vi "AutoSteerAngle.vi"(4 "CurrentSteerAngle":dbl, 6 "CurrentDirection":dbl, 8 "Ycurrent":dbl, 9 "Xcurrent":dbl, 10 "Ywaypoint":dbl, 11 "Xwaypoint":dbl) -> (2 "NewSteerAngle":dbl)   [LabVIEW 2012]
doc: "This VI calculates steering angle from current robot position to next waypoint."
uses:
  <vilib>/addons/control/pid/pid.llb/PID (DBL).vi
  <vilib>/addons/control/pid/NI_PID_pid.lvlib
panel:
  in  "reinitialize? (F)":bool
  out "reranged":dbl
  out "SetpointCommand":dbl
  out "Waveform Chart 2":cluster{dbl, dbl}(graph)
  out "output range":cluster{"output high":dbl, "output low":dbl}={"output high"=100.0, "output low"=-100.0} {"output low" format="%.2f"; "output high" format="%.2f"}
  out "PID gains":T1={"proportional gain (Kc)"=20.0, "integral time (Ti, min)"=0.008, "derivative time (Td, min)"=0.001} {"derivative time (Td, min)" step=1e-05 format="%.5f"; "integral time (Ti, min)" step=0.0001 format="%.4f"; "proportional gain (Kc)" step=0.001 format="%.4f"}
  out "Waveform Chart":cluster{dbl, "CurrentDirection":dbl}(graph)
  out "towaypoint":dbl
  # "This Vi calculates sttering angle \nfrom current position to \nnext waypoint"
  # "0.120\n1.600\n0000"
  # "in degreees"
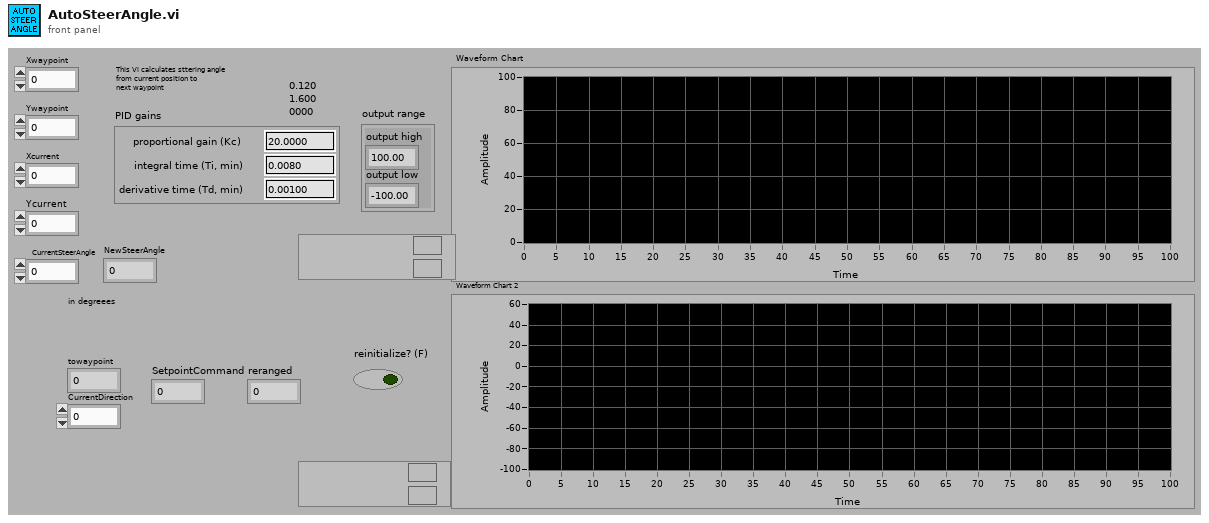
[diagram p1: front panel]
types:
  T1 = cluster{"proportional gain (Kc)":dbl, "integral time (Ti, min)":dbl, "derivative time (Td, min)":dbl}
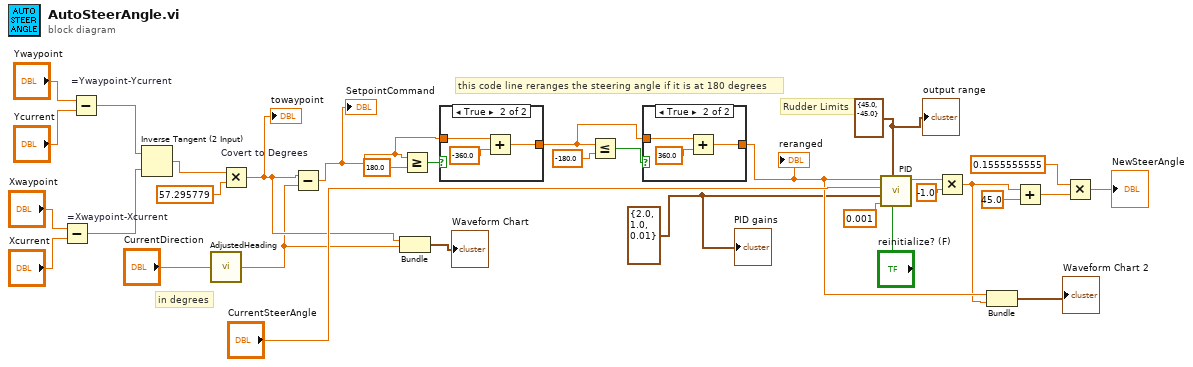
[diagram p0: block diagram]
diagram:
  w7 = T1 {"proportional gain (Kc)"=2.0, "integral time (Ti, min)"=1.0, "derivative time (Td, min)"=0.01} ("PID gains")
  w21 = cluster{"output high":dbl, "output low":dbl} {"output high"=45.0, "output low"=-45.0} ("output range")
  # "this code line reranges the steering angle if it is at 180 degrees"
  # "Rudder Limits"
  # "in degrees"
  n1 = Subtract "=Xwaypoint-Xcurrent"(x="Xwaypoint", y="Xcurrent") -> (x-y=w27:dbl)
  n2 = Subtract "=Ywaypoint-Ycurrent"(x="Ywaypoint", y="Ycurrent") -> (x-y=w28:dbl)
  n3 = Inverse Tangent (2 Input)(1:w27, 2:w28) -> (0:w25:dbl)
  n4 = call "AdjustedHeading.vi"("Heading In"="CurrentDirection") -> ("Heading Out"=w1:dbl)
  n5 = Multiply "Covert to Degrees"(x=w25, y=57.295779) -> (x*y=w13:dbl)
  "towaypoint" <- w13
  n6 = Subtract(x=w13, y=w1) -> (x-y=w17:dbl)
  "SetpointCommand" <- w17
  n7 = Bundle(w13, "Heading Out"=w1) -> (→"Waveform Chart":cluster{dbl, "Heading Out":dbl})  [unwired: 1 in]
  n8 = Greater Or Equal?(x=w17, y=180.0) -> (x >= y?=w18:bool)
  n9 = case shown="True" w18 {
    tunnel: w17 -> [w33 w36]
    tunnel: [w33 w34] -> w14
    frame False {
    }
    frame True {
      n10 = Add(x=w36, y=-360.0) -> (x+y=w34:dbl)
    }
  }
  n11 = Less Or Equal?(x=w14, y=-180.0) -> (x <= y?=w15:bool)
  n12 = case shown="True" w15 {
    tunnel: w14 -> [w37 w40]
    tunnel: [w37 w38] -> w10
    frame False {
    }
    frame True {
      n13 = Add(x=w40, y=360.0) -> (x+y=w38:dbl)
    }
  }
  "reranged" <- w10
  n14 = call-poly <vilib>:"PID.vi"("reinitialize? (F)"="reinitialize? (F)", "output range"=w21, "dt (s)"=0.001, "PID gains"=w7, "process variable"="CurrentSteerAngle", "setpoint"=w10) -> ("output"=w22:dbl)  [unwired: 4 in, 1 out]
  n15 = Multiply(x=w22, y=-1.0) -> (x*y=w5:dbl)
  n16 = Bundle(w10, w5) -> (→"Waveform Chart 2":cluster{dbl, dbl})  [unwired: 1 in]
  n17 = Add(x=w5, y=45.0) -> (x+y=w4:dbl)
  n18 = Multiply(x=0.1555555555, y=w4) -> (x*y=→"NewSteerAngle":dbl)
  "PID gains" <- w7
  "output range" <- w21
